vi "OP10_CRIMP_10_53_25_AM.vi"() -> ()   [LabVIEW 2020]
panel:
  in  "OP10_CRIMP":T1
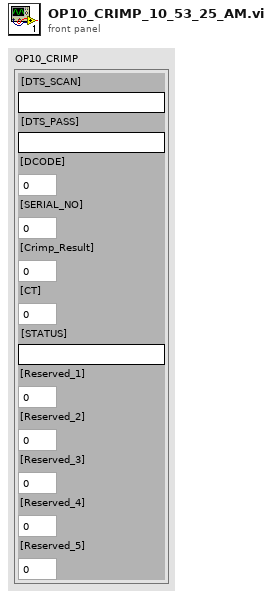
[diagram p1: front panel]
types:
  T1 = cluster{"[DTS_SCAN]":string, "[DTS_PASS]":string, "[DCODE]":dbl, "[SERIAL_NO]":dbl, "[Crimp_Result]":dbl, "[CT]":dbl, "[STATUS]":string, "[Reserved_1]":dbl, "[Reserved_2]":dbl, "[Reserved_3]":dbl, "[Reserved_4]":dbl, "[Reserved_5]":dbl}
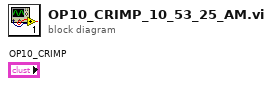
[diagram p0: block diagram]
diagram:
